vi "更新全局变量.vi"() -> ()   [LabVIEW 2016, in "update.lvlib"]
uses:
  update.lvlib
  <vilib>/FTP/ftp2.llb/FTP File Info.ctl
  <vilib>/FTP/NI_FTP.lvlib
panel:
  out "已下载大小":i64
  out "滑动杆":dbl(slide) scale=0.0..100.0
  out "path info":T1={"type"=enum."link", "permissions"="", "owner"="", "group"="", "size"=0, "date"="", "name"="", "link name"=""} caption="路径信息"
  out "command":string caption="命令"
  out "last status string":string caption="最近状态字符串"
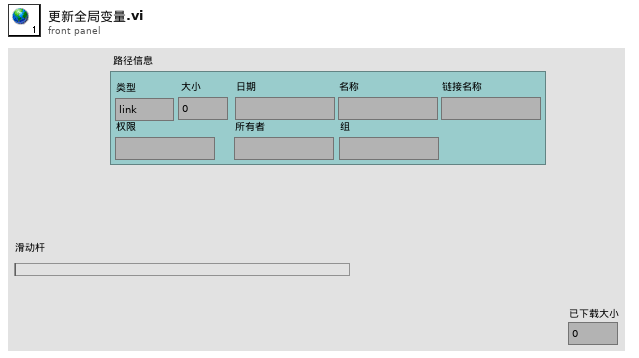
[diagram p1: front panel]
types:
  T1 = typedef "NI_FTP.lvlib/FTP File Info.ctl" = cluster{"type":enum16{"unknown", "file", "dir", "link"}, "permissions":string, "owner":string, "group":string, "size":i32, "date":string, "name":string, "link name":string}
diagram:
